vi "ANALOG INPUT.vi"() -> ()   [LabVIEW 2021]
uses:
  <vilib>/Instr/_visa.llb/VISA Configure Serial Port (Instr).vi
panel:
  out "Meter":dbl(knob) scale=0.0..1023.0
  out "Tank":dbl(slide) scale=0.0..1023.0
  out "String":string
  in  "VISA resource name":refnum<visa-resource-name>
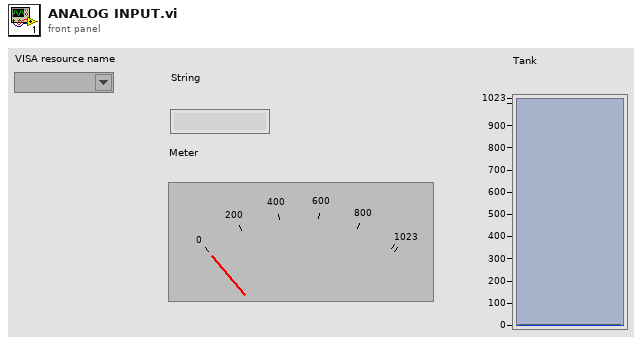
[diagram p1: front panel]
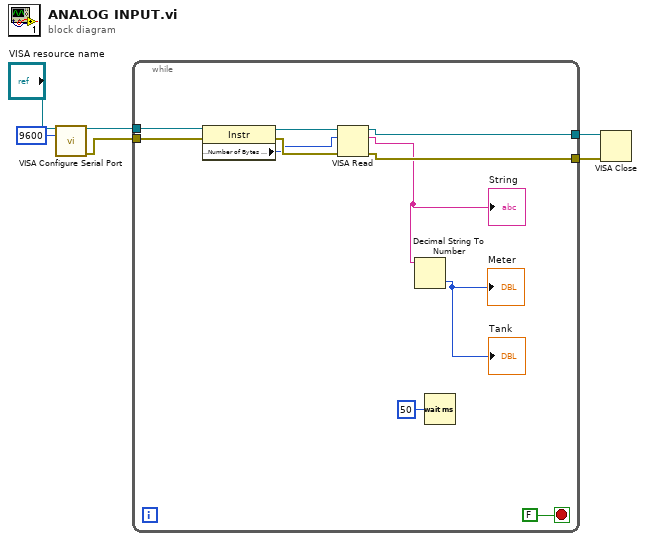
[diagram p0: block diagram]
diagram:
  n1 = call-poly "VISA Configure Serial Port"("VISA resource name"="VISA resource name", "baud rate (9600)"=u32 9600) -> ("VISA resource name out"=w6:refnum<visa-resource-name>, "error out"=w4:errorcluster)  [unwired: 12 in]
  n2 = while {
    tunnel: w6 -> [w17]
    tunnel: [w15] -> w5
    tunnel: w4 -> [w14]
    tunnel: [w12] -> w3
    stop <- FALSE stop-if-true
    n3 = property class="Instr"(reference=w17, error in=w14) -> (reference out=w16:refnum<visa-resource-name>, error out=w13:errorcluster, "Serial Settings:Number of Bytes at Serial Port"=w11:u32)
    n4 = VISA Read(VISA resource name=w16, byte count=w11, error in (no error)=w13) -> (VISA resource name out=w15:refnum<visa-resource-name>, read buffer=w8:string, error out=w12:errorcluster)  [unwired: 1 out]
    "String" <- w8
    n5 = Decimal String To Number(string=w8) -> (number=→"Tank" →"Meter":i32)  [unwired: 2 in, 1 out]
    n6 = Wait (ms)(milliseconds to wait=u32 50) -> ()  [unwired: 1 out]
  }
  n7 = VISA Close(VISA resource name=w5, error in (no error)=w3) -> ()  [unwired: 1 out]
